vi "Untitled 4.vi"() -> ()   [LabVIEW 2013]
panel:
  out "回復訊息":string
  in  "Enum":T1(ring)=enum."雷射觸發"
  in  "OK Button":bool
  in  "STOP":bool
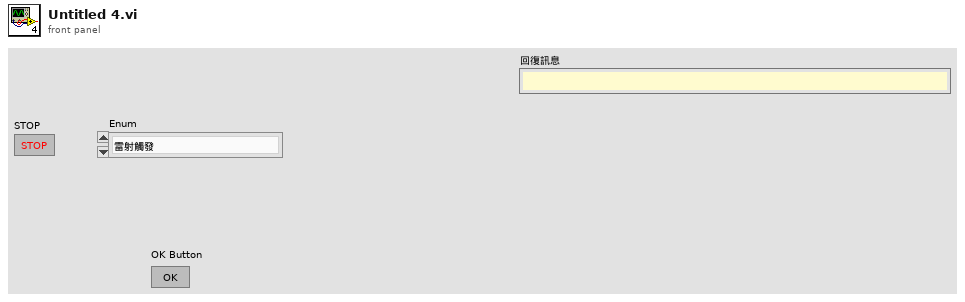
[diagram p1: front panel]
types:
  T1 = enum16{"RS232_Init ", "雷射準備訊號", "雷射觸發", "RS232_Close", "讀出雷射XY座標值", "寫入雷射XY座標值", "請求程式編號prog"}
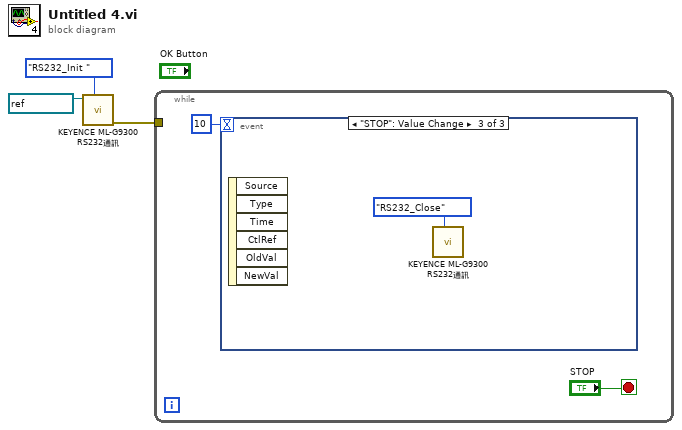
[diagram p0: block diagram]
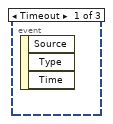
[diagram p2: hidden frame]
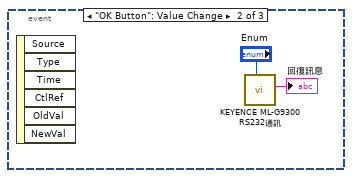
[diagram p3: hidden frame]
diagram:
  n1 = call "KEYENCE ML-G9300 RS232通訊.vi"("Enum"=T1."RS232_Init ", "VISA resource name"=refnum<visa-resource-name> "COM1") -> ("error out"=w1:errorcluster)  [unwired: 7 in, 2 out]
  n2 = while {
    tunnel: w1 -> [_]
    stop <- "STOP" stop-if-true
    n3 = event shown="[2] \"STOP\": Value Change" {
      selector: _ -> [_ _ _]
      dyn-events: _ -> [_ _ _]
      timeout: 10 -> [_ _ _]
      event Timeout {
        n4 = event-data() -> ()  [unwired: 1 in, 3 out]
      }
      event "OK Button": Value Change {
        n5 = event-data() -> ()  [unwired: 1 in, 6 out]
        n6 = call "KEYENCE ML-G9300 RS232通訊.vi"("Enum"="Enum") -> ("回復訊息"=→"回復訊息":string)  [unwired: 8 in, 2 out]
      }
      event "STOP": Value Change {
        n7 = event-data() -> ()  [unwired: 1 in, 6 out]
        n8 = call "KEYENCE ML-G9300 RS232通訊.vi"("Enum"=T1."RS232_Close") -> ()  [unwired: 8 in, 3 out]
      }
    }
  }
